vi "NM SAVE MEI.vi"(4 "WT CODE":i32, 6 "Slide in":refnum<vi>, 7 "NM?":bool, 8 "error out IN":errorcluster, 9 "ItemNames":string[][](array[string]), 10 "Array vf":bool[][][](array[boolean]), 11 "Array MEMO":string[][][](array[string])) -> (0 "error out":errorcluster)   [LabVIEW 2019]
uses:
  <vilib>/addons/database/NI_Database_API.lvlib
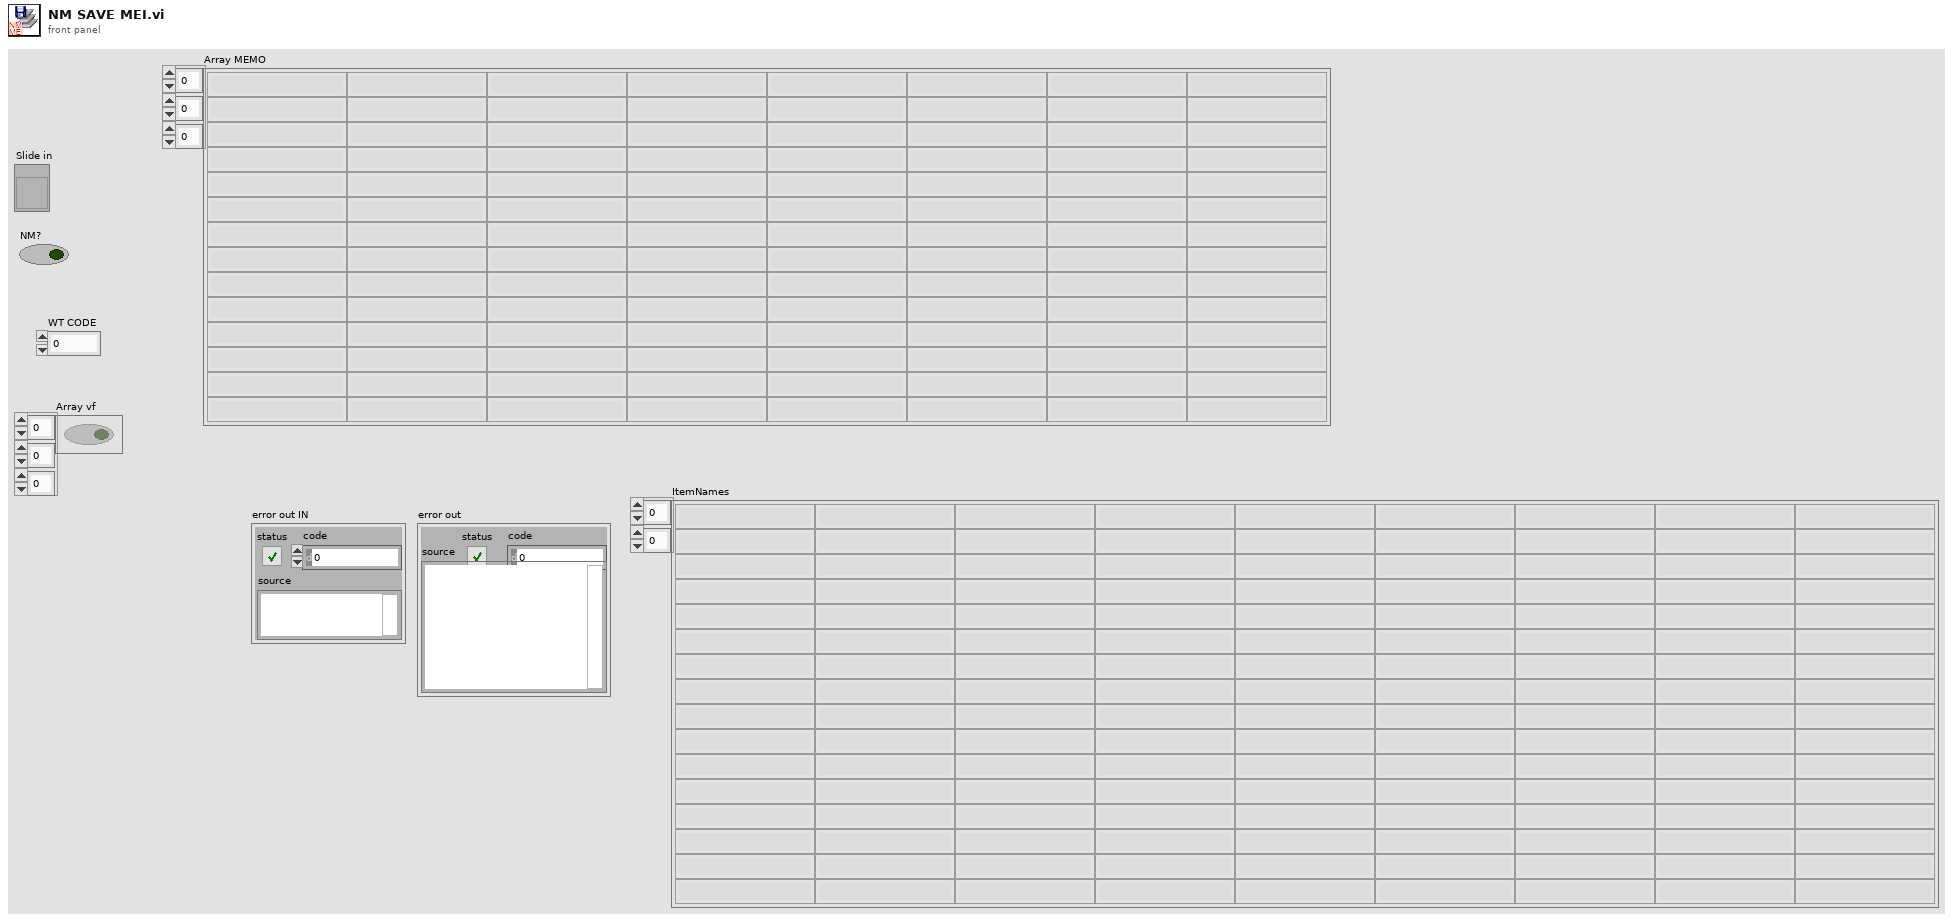
[diagram p1: front panel]
types:
  T1 = cluster{"Array of elements":cluster{"String":string, "variant":variant}[], "Single element":cluster{"String":string, "variant":variant}, "enque at\nopposite end (F)":bool, "no replications (F)":bool}
  T2 = typedef "NI_Database_API.lvlib/Conn ObjectReference.ctl" = refnum<k1>
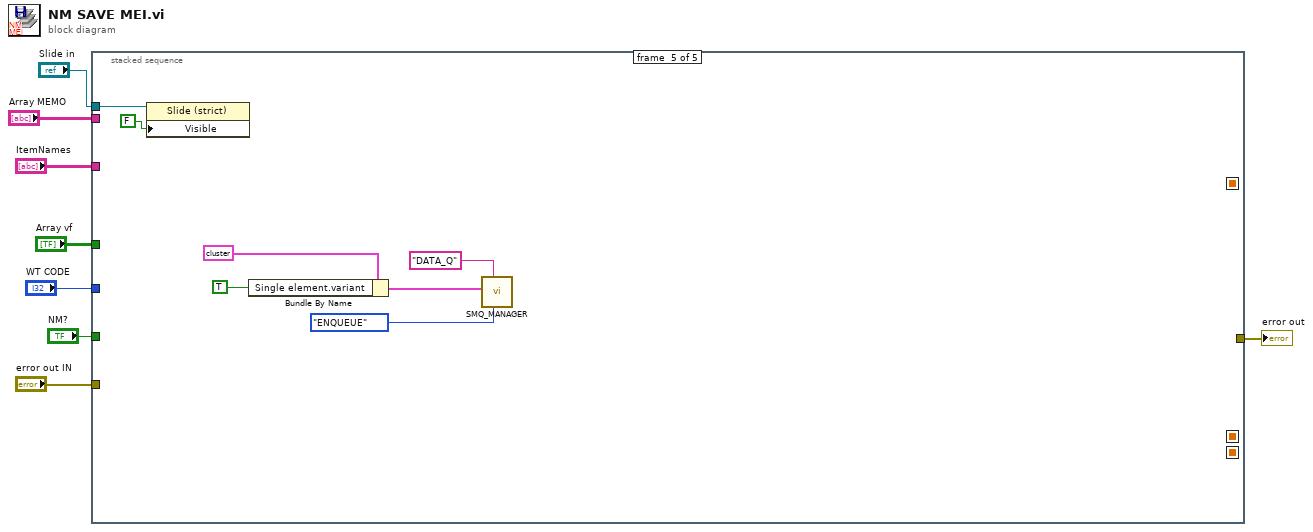
[diagram p0: block diagram]
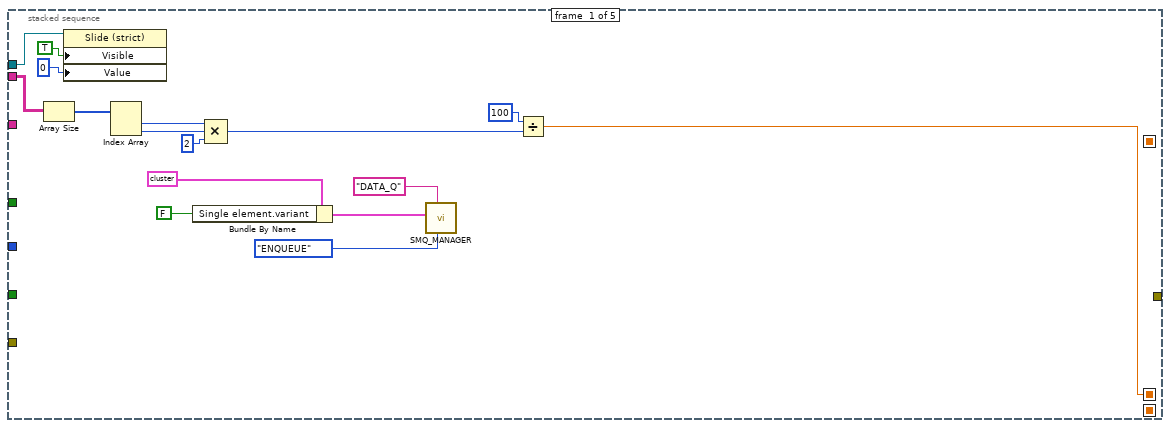
[diagram p2: hidden frame]
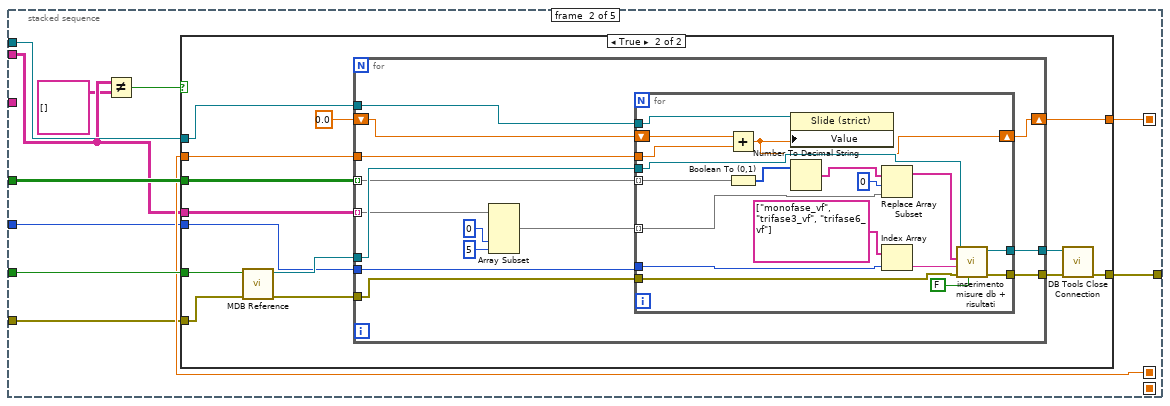
[diagram p3: hidden frame]
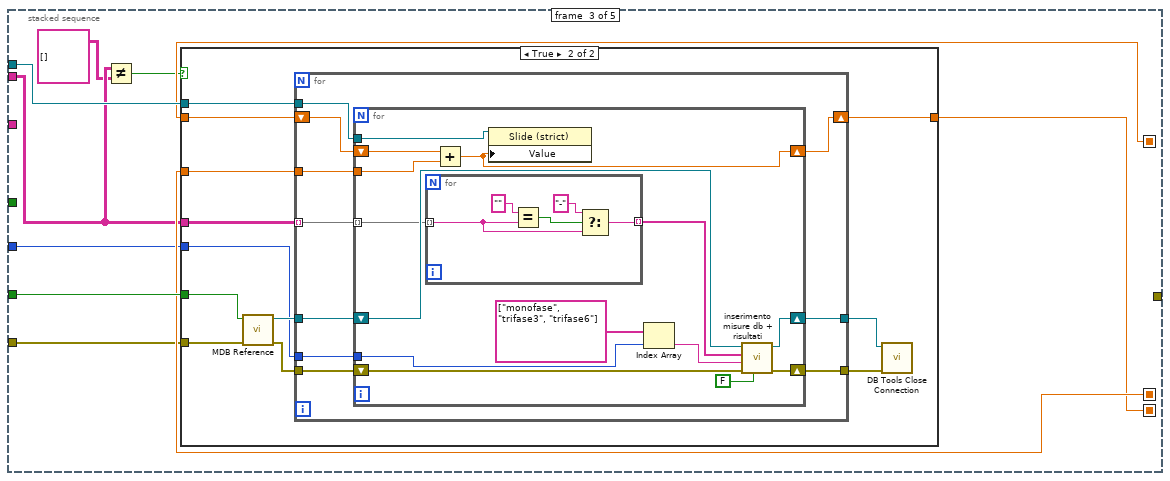
[diagram p5: hidden frame]
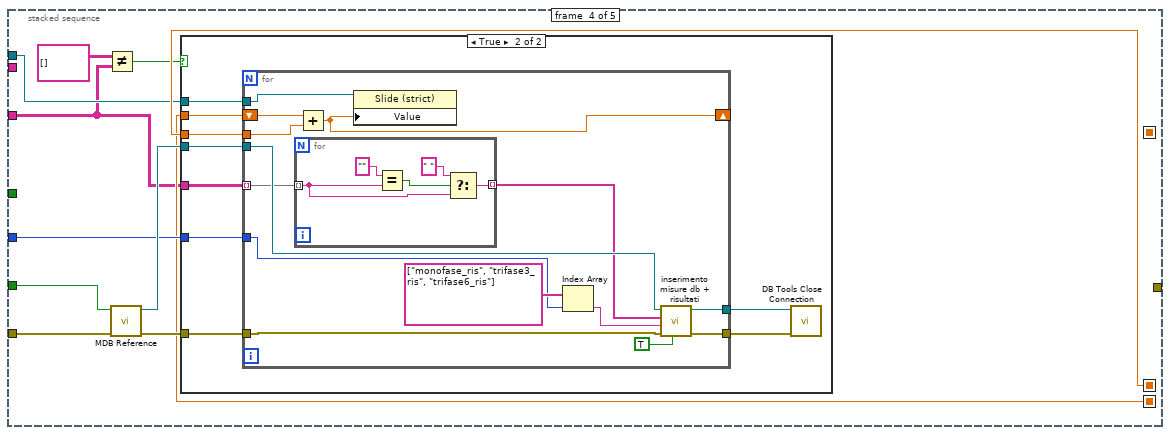
[diagram p7: hidden frame]
diagram:
  n1 = stacked-sequence {
    seq-local: [w12 _ _ _ _] -> [_ w33 w92 w143 _]
    seq-local: [_ w29 _ _ _] -> [_ _ w88 _ _]
    seq-local: [_ _ w87 _ _] -> [_ _ _ w139 _]
    tunnel: "Array MEMO" -> [w19 w27 w86 _ _]
    tunnel: "Array vf" -> [_ w34 _ _ _]
    tunnel: "NM?" -> [_ w35 w93 w146 _]
    tunnel: [_ w28 _ _ _] -> w7
    tunnel: "ItemNames" -> [_ _ _ w138 _]
    tunnel: "Slide in" -> [w10 w32 w91 w142 w175]
    tunnel: "error out IN" -> [_ w31 w90 w141 _]
    tunnel: "WT CODE" -> [_ w30 w89 w140 _]
    frame #0 {
      n2 = Array Size(array=w19) -> (size(s)=w18:i32[])
      n3 = property on="Property Node" class="Slide (strict)"(reference=w10, "Visible"=TRUE, "Value"=u8 0) -> ()  [unwired: 1 in, 2 out]
      n4 = Index Array(array=w18) -> (element #1=w17:i32, element #2=w16:i32)  [unwired: 2 in]
      n5 = Bundle By Name(cluster=T1 {"Array of elements"=[], "Single element"={"String"="SEND MAIN2?", "variant"=variant}, "enque at\nopposite end (F)"=FALSE, "no replications (F)"=FALSE} ("Enqueue cluster"), "Single element.variant"=FALSE) -> (w20:T1)
      n6 = Compound Arithmetic op=MULTIPLY(w17, w16, 2 ("value")) -> (w13:i32)
      n7 = call <userlib>:"SMQ_MANAGER.vi"("Function"=enum16{"INITIALIZE", "ENQUEUE", "STOP ALL"}."ENQUEUE", "Queue name"="DATA_Q", "Enqueue cluster"=w20) -> ()  [unwired: 8 in, 1 out]
      n8 = Divide(x=100, y=w13) -> (x/y=w12:dbl)
    }
    frame #1 {
      n9 = Not Equal?(x=w27, y=string[][][] []) -> (x != y?=w25:bool)
      n10 = case shown="True" w25 {
        tunnel: w35 -> [_ w51]
        tunnel: w34 -> [_ w47]
        tunnel: w33 -> [w37 w45]
        tunnel: w32 -> [_ w44]
        tunnel: w31 -> [w36 w43]
        tunnel: w30 -> [_ w42]
        tunnel: [w37 w40] -> w29
        tunnel: [w36 w39] -> w28
        tunnel: w27 -> [_ w38]
        frame False {
        }
        frame True {
          n11 = call "MDB Reference.vi"("error in (no error)"=w43, "Collaudi T/motori F"=w51) -> ("error out"=w46:errorcluster, "Refnum out"=w50:T2)  [unwired: 7 in, 1 out]
          n12 = for {
            tunnel: w50 -> [w65]
            tunnel: [w64] -> w49
            tunnel: [w63] -> w48
            tunnel: w47 -> [w62] mode=indexing
            tunnel: w38 -> [w60] mode=indexing
            tunnel: w46 -> [w57]
            tunnel: w45 -> [w56]
            tunnel: w44 -> [w55]
            tunnel: w42 -> [w54]
            shift-right: [w52] -> w40
            shift-left: 0.0 -> [w53]
            n13 = Array Subset "Array Subset"(array=w60, index (col)=0 ("index"), length (col)=5 ("length")) -> (w58:string[][])  [unwired: 2 in]
            n14 = for {
              tunnel: [w80] -> w63
              tunnel: w65 -> [w83]
              tunnel: [w82] -> w64
              tunnel: w62 -> [w70] mode=indexing
              tunnel: w58 -> [w78] mode=indexing
              tunnel: w57 -> [w76]
              tunnel: w56 -> [w75]
              tunnel: w55 -> [w68]
              tunnel: w54 -> [w72]
              shift-right: [w66] -> w52
              shift-left: w53 -> [w67]
              n15 = Add(x=w67, y=w75) -> (x+y=w66:dbl)
              n16 = Boolean To (0,1)(Boolean=w70) -> (0, 1=w71:i16[])
              n17 = property on="Property Node" class="Slide (strict)"(reference=w68, "Value"=w66) -> ()  [unwired: 1 in, 2 out]
              n18 = Number To Decimal String(number=w71) -> (decimal integer string=w69:string[])  [unwired: 1 out]
              n19 = Replace Array Subset(array=w69, new element=w78, index=0) -> (w77:string[])
              n20 = Index Array(array=string[] ["monofase_vf", "trifase3_vf", "trifase6_vf"], index=w72) -> (element=w73:string)
              n21 = call "inserimento misure db + risultati.vi"("Risultati?"=FALSE, "error out in"=w76, "nome tabella"=w73, "Risultati"=w77, "connection reference"=w83) -> ("error out"=w80:errorcluster, "connection reference out"=w82:T2)  [unwired: 4 in, 1 out]
            }
          }
          n22 = call <vilib>:"DB Tools Close Connection.vi"("error in (no error)"=w48, "connection reference"=w49) -> ("error out"=w39:errorcluster)  [unwired: 5 in]
        }
      }
    }
    frame #2 {
      n23 = Not Equal?(x=w86, y=string[][][] []) -> (x != y?=w84:bool)
      n24 = case shown="True" w84 {
        tunnel: w93 -> [_ w106]
        tunnel: w86 -> [_ w101]
        tunnel: w92 -> [_ w100]
        tunnel: w91 -> [_ w99]
        tunnel: w90 -> [_ w98]
        tunnel: w89 -> [_ w97]
        tunnel: w88 -> [w94 w96]
        tunnel: [w94 w95] -> w87
        frame False {
        }
        frame True {
          n25 = call "MDB Reference.vi"("error in (no error)"=w98, "Collaudi T/motori F"=w106) -> ("error out"=w102:errorcluster, "Refnum out"=w105:T2)  [unwired: 7 in, 1 out]
          n26 = for {
            tunnel: w105 -> [w116]
            tunnel: w101 -> [w115] mode=indexing
            tunnel: [w114] -> w104
            tunnel: [w113] -> w103
            tunnel: w102 -> [w112]
            tunnel: w100 -> [w111]
            tunnel: w99 -> [w110]
            tunnel: w97 -> [w109]
            shift-right: [w107] -> w95
            shift-left: w96 -> [w108]
            n27 = for {
              tunnel: w115 -> [w125] mode=indexing
              shift-right: [w129] -> w114
              shift-left: w116 -> [w130]
              shift-right: [w123] -> w113
              shift-left: w112 -> [w127]
              tunnel: w111 -> [w126]
              tunnel: w110 -> [w119]
              tunnel: w109 -> [w121]
              shift-right: [w117] -> w107
              shift-left: w108 -> [w118]
              n28 = for {
                tunnel: w125 -> [w133] mode=indexing
                tunnel: [w131] -> w124 mode=indexing
                n29 = Equal?(x="", y=w133) -> (x = y?=w134:bool)
                n30 = Select(t="-", s=w134, f=w133) -> (s? t:f=w131:string)
              }
              n31 = Add(x=w118, y=w126) -> (x+y=w117:dbl)
              n32 = property on="Property Node" class="Slide (strict)"(reference=w119, "Value"=w117) -> ()  [unwired: 1 in, 2 out]
              n33 = Index Array(array=string[] ["monofase", "trifase3", "trifase6"], index=w121) -> (element=w120:string)
              n34 = call "inserimento misure db + risultati.vi"("Risultati?"=FALSE, "error out in"=w127, "nome tabella"=w120, "Risultati"=w124, "connection reference"=w130) -> ("error out"=w123:errorcluster, "connection reference out"=w129:T2)  [unwired: 4 in, 1 out]
            }
          }
          n35 = call <vilib>:"DB Tools Close Connection.vi"("error in (no error)"=w103, "connection reference"=w104) -> ()  [unwired: 5 in, 1 out]
        }
      }
    }
    frame #3 {
      n36 = Not Equal?(x=string[][] [], y=w138) -> (x != y?=w136:bool)
      n37 = call "MDB Reference.vi"("error in (no error)"=w141, "Collaudi T/motori F"=w146) -> ("error out"=w144:errorcluster, "Refnum out"=w145:T2)  [unwired: 7 in, 1 out]
      n38 = case shown="True" w136 {
        tunnel: w145 -> [_ w155]
        tunnel: w144 -> [_ w152]
        tunnel: w143 -> [_ w151]
        tunnel: w138 -> [_ w150]
        tunnel: w142 -> [_ w149]
        tunnel: w140 -> [_ w148]
        tunnel: w139 -> [_ w147]
        frame False {
        }
        frame True {
          n39 = for {
            tunnel: w155 -> [w169]
            tunnel: w150 -> [w163] mode=indexing
            tunnel: [w168] -> w154
            tunnel: [w166] -> w153
            tunnel: w152 -> [w165]
            tunnel: w151 -> [w164]
            tunnel: w149 -> [w158]
            tunnel: w148 -> [w160]
            shift-right: [w156] -> _
            shift-left: w147 -> [w157]
            n40 = for {
              tunnel: w163 -> [w172] mode=indexing
              tunnel: [w170] -> w162 mode=indexing
              n41 = Equal?(x="", y=w172) -> (x = y?=w173:bool)
              n42 = Select(t=" ", s=w173, f=w172) -> (s? t:f=w170:string)
            }
            n43 = Add(x=w157, y=w164) -> (x+y=w156:dbl)
            n44 = property on="Property Node" class="Slide (strict)"(reference=w158, "Value"=w156) -> ()  [unwired: 1 in, 2 out]
            n45 = Index Array(array=string[] ["monofase_ris", "trifase3_ris", "trifase6_ris"], index=w160) -> (element=w159:string)
            n46 = call "inserimento misure db + risultati.vi"("Risultati?"=TRUE, "error out in"=w165, "nome tabella"=w159, "Risultati"=w162, "connection reference"=w169) -> ("error out"=w166:errorcluster, "connection reference out"=w168:T2)  [unwired: 4 in, 1 out]
          }
          n47 = call <vilib>:"DB Tools Close Connection.vi"("error in (no error)"=w153, "connection reference"=w154) -> ()  [unwired: 5 in, 1 out]
        }
      }
    }
    frame #4 {
      n48 = property on="Property Node" class="Slide (strict)"(reference=w175, "Visible"=FALSE) -> ()  [unwired: 1 in, 2 out]
      n49 = Bundle By Name(cluster=T1 {"Array of elements"=[], "Single element"={"String"="SEND MAIN2?", "variant"=variant}, "enque at\nopposite end (F)"=FALSE, "no replications (F)"=FALSE} ("Enqueue cluster"), "Single element.variant"=TRUE) -> (w177:T1)
      n50 = call <userlib>:"SMQ_MANAGER.vi"("Function"=enum16{"INITIALIZE", "ENQUEUE", "STOP ALL"}."ENQUEUE", "Queue name"="DATA_Q", "Enqueue cluster"=w177) -> ()  [unwired: 8 in, 1 out]
    }
  }
  "error out" <- w7
